vi "Data Get Double (Polymorphic).vi"   [LabVIEW 2012]
uses:
  <vilib>/MDSplus/Library/MDSplus.lvlib
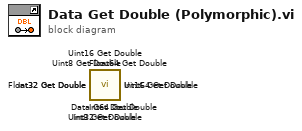
[diagram p0: block diagram]
diagram:
  n1 = call <vilib>:"Data Get Double.vi"() -> ()  [unwired: 9 in, 3 out]
  n2 = call <vilib>:"Float64 Get Double.vi"() -> ()  [unwired: 9 in, 3 out]
  n3 = call <vilib>:"Float32 Get Double.vi"() -> ()  [unwired: 9 in, 3 out]
  n4 = call <vilib>:"Uint64 Get Double.vi"() -> ()  [unwired: 9 in, 3 out]
  n5 = call <vilib>:"Uint32 Get Double.vi"() -> ()  [unwired: 9 in, 3 out]
  n6 = call <vilib>:"Uint16 Get Double.vi"() -> ()  [unwired: 9 in, 3 out]
  n7 = call <vilib>:"Uint8 Get Double.vi"() -> ()  [unwired: 9 in, 3 out]
  n8 = call <vilib>:"Int64 Get Double.vi"() -> ()  [unwired: 9 in, 3 out]
  n9 = call <vilib>:"Int32 Get Double.vi"() -> ()  [unwired: 9 in, 3 out]
  n10 = call <vilib>:"Int16 Get Double.vi"() -> ()  [unwired: 9 in, 3 out]
  n11 = call <vilib>:"Int8 Get Double.vi"() -> ()  [unwired: 9 in, 3 out]
